vi "Create Initiation Keys.vi"(8 "error in":errorcluster, 11 "srp":T1) -> (0 "error out":errorcluster, 2 "PUblicKeyA":u8[](array[numeric]), 3 "srp":T1)   [LabVIEW 2016, in "SRP.lvlib"]
uses:
  <vilib>/addons/InsightCM/SRP/SRP.lvlib
  <vilib>/addons/InsightCM/SRP/controls/DVR_data.ctl
  <vilib>/addons/InsightCM/SRP/controls/data.ctl
  <vilib>/addons/InsightCM/SRP/libraries/win32Urelease/brsrp.dll
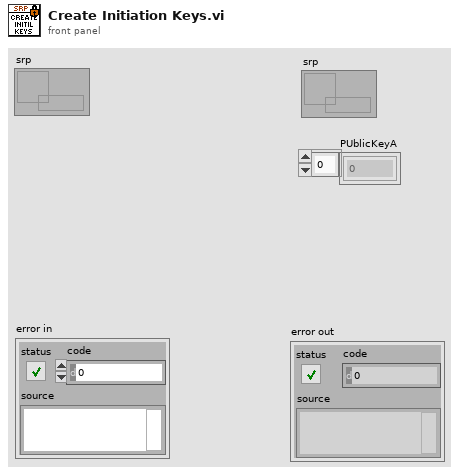
[diagram p1: front panel]
types:
  T1 = typedef "SRP.lvlib/DVR_data.ctl" = refnum<data-value>
  T2 = typedef "SRP.lvlib/data.ctl" = cluster{"SessionKey":u8[], "ClientHash":u8[], "PublicKeyA":u8[], "PrivateKeyA":u8[]}
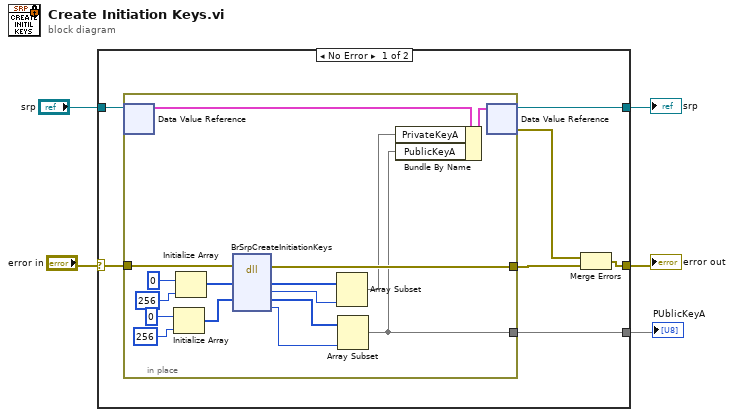
[diagram p0: block diagram]
diagram:
  n1 = case shown="No Error" "error in" {
    selector: "error in" -> [w8 w30]
    tunnel: [w10 w30] -> w5
    tunnel: "srp" -> [w12 w29]
    tunnel: [w11 w29] -> w2
    tunnel: [w6 _] -> w1
    frame No Error {
      n2 = in-place {
        in-place-border: w8 -> [w23]
        in-place-border: [w22] -> w7
        in-place-border: [w15] -> w6
        n3 = in-place-dvr #1(w12) -> (w28:T2)  [unwired: 1 out]
        n4 = Initialize Array(u8 0, 256 ("dimension size")) -> (w21:u8[])
        n5 = Initialize Array(u8 0, 256 ("dimension size")) -> (w18:u8[])
        n6 = dll-call lib="C:/Program Files (x86)/National Instruments/LabVIEW 2016/vi.lib/addons/InsightCM/SRP/libraries/win32Urelease/brsrp.*" fn="BrSrpCreateInitiationKeys"(error in=w23, "privateKeyA"=w18, "publicKeyA"=w21) -> (error out=w22:errorcluster, "privateKeyA"=w17:u8[], "length_privateKeyA"=w14:u32, "publicKeyA"=w24:u8[], "length_PublicKeyA"=w13:u32)  [unwired: 5 in, 1 out]
        n7 = Array Subset(array=w17, length=w14) -> (w16:u8[])  [unwired: 1 in]
        n8 = Array Subset(array=w24, length=w13) -> (w15:u8[])  [unwired: 1 in]
        n9 = Bundle By Name(cluster=w28, "PrivateKeyA"=w16, "PublicKeyA"=w15) -> (w27:T2)
        n10 = in-place-dvr #1(w27) -> (w11:T1, w9:errorcluster)
      }
      n11 = Merge Errors(w9, w7) -> (w10:errorcluster)
    }
    frame Error {
    }
  }
  "error out" <- w5
  "srp" <- w2
  "PUblicKeyA" <- w1
